vi "example test.vi"() -> ()   [LabVIEW 2013, in "processing plugin tests.lvlib"]
uses:
  processing plugin tests.lvlib
  module/configuration/tag bus processing plugin module configuration.lvclass
  <vilib>/NI/Tag Bus Module Framework/channel/channel classification.ctl
  <vilib>/NI/Tag Bus/tag/Data Type.ctl
  module/execution/tag bus processing plugin module.lvclass
  module/configuration/processing channels.ctl
  <vilib>/NI/Tag Bus Module Framework/channel/TBM channel.lvclass
  <vilib>/NI/Tag Bus/dictionary/data dictionary.lvclass/data dictionary.ctl
  <vilib>/NI/Tag Bus/dictionary/lookup polymorphs/locate double.vi
  <vilib>/NI/Tag Bus/table/data polymorphs/write one/write Double.vi
  <vilib>/NI/Tag Bus/table/data polymorphs/read one/read Double.vi
  <vilib>/NI/Tag Bus/dictionary/search/find data index.vi
  <vilib>/NI/Tag Bus/dictionary/search/search string list.vi
  <vilib>/NI/Tag Bus/dictionary/tag not found.vi
  <vilib>/NI/Tag Bus/tag/tag descriptor.lvclass
  <vilib>/NI/Tag Bus/dictionary/data dictionary.lvclass
  <vilib>/NI/Tag Bus/table/data table.lvlib
panel:
  out "result":dbl
  out "param lookup error":errorcluster
  out "final error":errorcluster
  out "proc error":errorcluster
  out "output lookup error":errorcluster
  out "init error":errorcluster
  out "correct execution settings":bool
  out "serialization problem":errorcluster
  out "invalid configuration":errorcluster
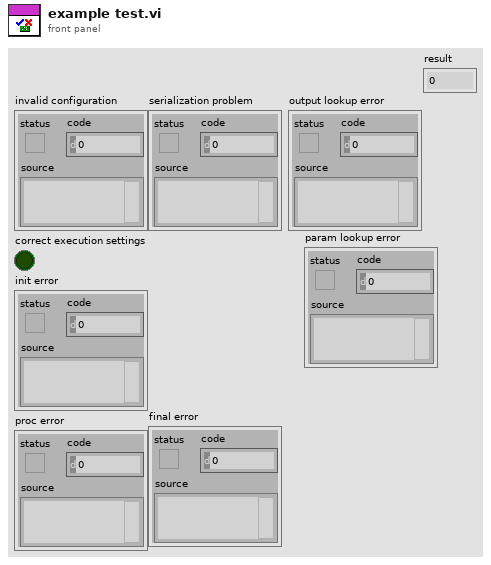
[diagram p1: front panel]
types:
  T1 = typedef "tag bus processing plugin module configuration.lvclass/processing channels.ctl" = cluster{"parameter":refnum<class "TBM channel.lvclass">, "result":refnum<class "TBM channel.lvclass">}
  T2 = typedef "TBM channel.lvclass/channel classification.ctl" = enum16{"input data", "output data", "processing parameter", "processing result"}
  T3 = typedef "tag bus.lvlib/tag descriptor.lvclass/Data Type.ctl" = enum16{"Double", "Single", "I64", "I32", "I16", "I8", "U64", "U32", "U16", "U8", "Boolean", "String", "Array of Double", "Array of Single", "Array of I64", "Array of I32", "Array of I16", "Array of I8", "Array of U64", "Array of U32", "Array of U16", "Array of U8", "Array of Boolean", "Array of String"}
  T4 = typedef "TBM channel.lvclass/data tables.ctl" = cluster{"input data":T5, "processing parameter":T5, "processing result":T5, "output data":T5}
  T5 = typedef "tag bus.lvlib/dictionary table pair.ctl" = cluster{"data dictionary":refnum<class "data dictionary.lvclass">, "data table":T6}
  T6 = typedef "tag bus.lvlib/data table.lvlib/data table.ctl" = cluster{"Double":dbl[], "Single":sgl[], "I64":i64[], "I32":i32[], "I16":i16[], "I8":i8[], "U64":u64[], "U32":u32[], "U16":u16[], "U8":u8[], "Boolean":bool[], "String":string[], "Array of Double":cluster{"DBL Array":dbl[]}[], "Array of Single":cluster{"SGL Array":sgl[]}[], "Array of I64":cluster{"I64 Array":i64[]}[], "Array of I32":cluster{"I32 Array":i32[]}[], "Array of I16":cluster{"I16 Array":i16[]}[], "Array of I8":cluster{"I8 Array":i8[]}[], "Array of U64":cluster{"U64 Array":u64[]}[], "Array of U32":cluster{"U32 Array":u32[]}[], "Array of U16":cluster{"U16 Array":u16[]}[], "Array of U8":cluster{"U8 Array":u8[]}[], "Array of Boolean":cluster{"Boolean Array":bool[]}[], "Array of String":cluster{"String Array":string[]}[]}
  T7 = typedef "TBM module execution interface.lvclass/execution settings.ctl" = cluster{"reads inputs":bool, "processes data":bool, "writes outputs":bool}
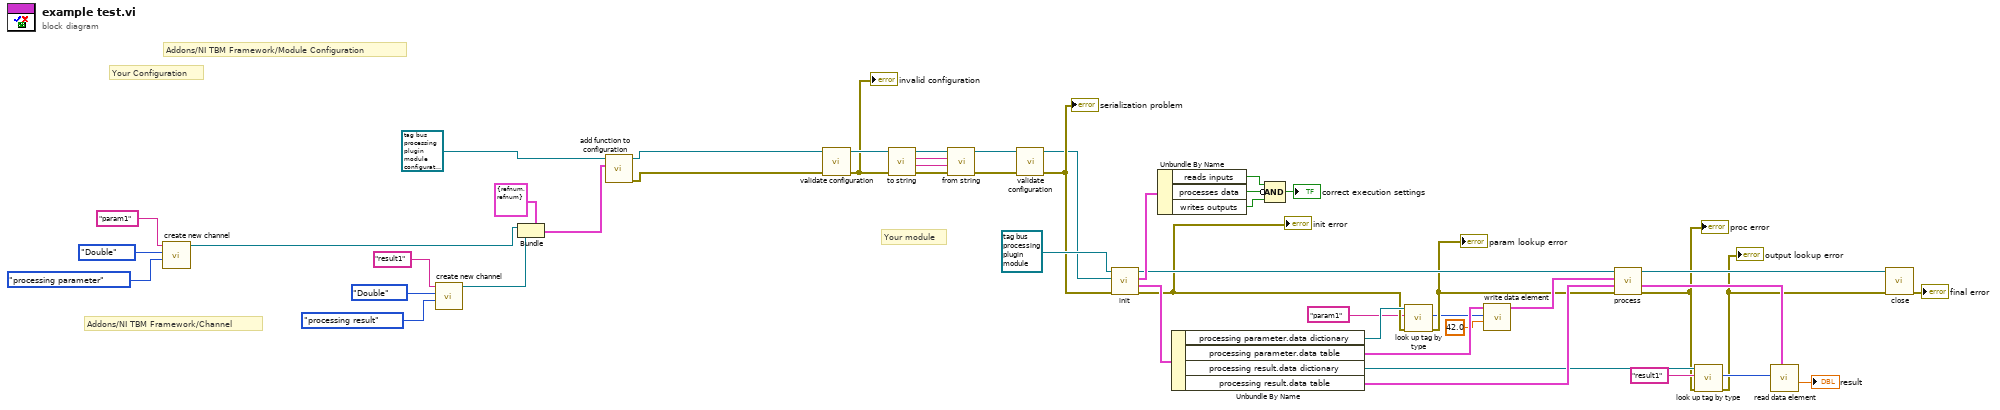
[diagram p0: block diagram]
diagram:
  # "Your module"
  # "Your Configuration"
  # "Addons/NI TBM Framework/Module Configuration"
  # "Addons/NI TBM Framework/Channel"
  n1 = call <vilib>:"create new channel.vi"("channel classification"=channel_classification."processing parameter", "data type"=Data_Type."Double", "channel name"="param1") -> ("channel"=w2:refnum<class "TBM channel.lvclass">)  [unwired: 8 in]
  n2 = call <vilib>:"create new channel.vi"("channel classification"=channel_classification."processing result", "data type"=Data_Type."Double", "channel name"="result1") -> ("channel"=w1:refnum<class "TBM channel.lvclass">)  [unwired: 8 in]
  n3 = Bundle(cluster=T1 {"parameter"=refnum, "result"=refnum} ("processing function"), "parameter"=w2, "result"=w1) -> (w3:T1)
  n4 = call "add function to configuration.vi"("processing function"=w3, "tag bus configurable plugin module configuration in"=refnum<class "tag bus processing plugin module configuration.lvclass"> refnum ("tag bus configurable plugin module configuration")) -> ("error out"=w5:errorcluster, "tag bus configurable plugin module configuration out"=w6:refnum<class "tag bus processing plugin module configuration.lvclass">)  [unwired: 8 in]
  n5 = call-dynamic "validate configuration.vi"("error in"=w5, "tag bus configurable plugin module configuration in"=w6) -> ("error out"=w42:errorcluster, "tag bus configurable plugin module configuration out"=w43:refnum<class "tag bus processing plugin module configuration.lvclass">)  [unwired: 8 in]
  "invalid configuration" <- w42
  n6 = call-dynamic "to string.vi"("error in"=w42, "tag bus configurable plugin module configuration in"=w43) -> ("error out"=w38:errorcluster, "data"=w39:string, "version"=w40:string, "tag bus configurable plugin module configuration out"=w41:refnum<class "tag bus processing plugin module configuration.lvclass">)  [unwired: 6 in]
  n7 = call-dynamic "from string.vi"("error in"=w38, "data"=w39, "version"=w40, "tag bus configurable plugin module configuration in"=w41) -> ("error out"=w36:errorcluster, "tag bus configurable plugin module configuration out"=w37:refnum<class "tag bus processing plugin module configuration.lvclass">)  [unwired: 6 in]
  n8 = call-dynamic "validate configuration.vi"("error in"=w36, "tag bus configurable plugin module configuration in"=w37) -> ("error out"=w34:errorcluster, "tag bus configurable plugin module configuration out"=w33:refnum<class "tag bus processing plugin module configuration.lvclass">)  [unwired: 8 in]
  "serialization problem" <- w34
  n9 = call-dynamic "init.vi"("error in"=w34, "TBM module configuration in"=w33, "tag bus configurable plugin module in"=refnum<class "tag bus processing plugin module.lvclass"> refnum ("tag bus configurable plugin module")) -> ("error out"=w19:errorcluster, "data allocations"=w27:T4, "execution settings"=w32:T7, "tag bus configurable plugin module out"=w25:refnum<class "tag bus processing plugin module.lvclass">)  [unwired: 5 in]
  "init error" <- w19
  n10 = Unbundle By Name(w32) -> ("reads inputs"=w29:bool, "processes data"=w31:bool, "writes outputs"=w30:bool)
  n11 = Unbundle By Name(w27) -> ("processing parameter.data dictionary"=w20:refnum<class "data dictionary.lvclass">, "processing parameter.data table"=w21:T6, "processing result.data dictionary"=w15:refnum<class "data dictionary.lvclass">, "processing result.data table"=w23:T6)
  n12 = Compound Arithmetic op=AND(w29, invert w31, w30) -> (→"correct execution settings":bool)
  n13 = call-poly <vilib>:"look up tag by type.vi"("error in"=w19, "name"="param1" ("channel name"), "data dictionary in"=w20) -> ("error out"=w18:errorcluster, "index"=w17:i32)  [unwired: 6 in, 1 out]
  "param lookup error" <- w18
  n14 = call-poly <vilib>:"write data element.vi"("value"=42.0, "index"=w17, "data table in"=w21) -> ("data table out"=w22:T6)  [unwired: 8 in]
  n15 = call-dynamic "process.vi"("error in"=w18, "result allocation"=w23, "data to process"=w22, "module in"=w25) -> ("error out"=w11:errorcluster, "result data"=w12:T6, "module out"=w24:refnum<class "tag bus processing plugin module.lvclass">)  [unwired: 4 in, 1 out]
  "proc error" <- w11
  n16 = call-poly <vilib>:"look up tag by type.vi"("error in"=w11, "name"="result1" ("channel name"), "data dictionary in"=w15) -> ("error out"=w9:errorcluster, "index"=w10:i32)  [unwired: 6 in, 1 out]
  "output lookup error" <- w9
  n17 = call-poly <vilib>:"read data element.vi"("index"=w10, "data table in"=w12) -> ("value"=→"result":dbl)  [unwired: 8 in, 1 out]
  n18 = call-dynamic "close.vi"("error in"=w9, "tag bus configurable plugin module in"=w24) -> ("error out"=→"final error":errorcluster)  [unwired: 9 in]
